vi "checkCalibrationChannel.vi"(8 "error in (no error)":errorcluster, 10 "Channel":T1, 11 "TEI9150 in":refnum<class "Tovey9150.lvclass">) -> (0 "error out":errorcluster, 2 "Items and Unit Numbers":string, 3 "TEI9150 out":refnum<class "Tovey9150.lvclass">)   [LabVIEW 2015, in "Tovey9150.lvclass"]
uses:
  Tovey9150.lvclass
  ToveyChannels.ctl
  Tovey9150.lvclass/Tovey9150.ctl
  <userlib>/Common/SerialProtocols/SerialCommunicator/SerialCommunicator.lvclass
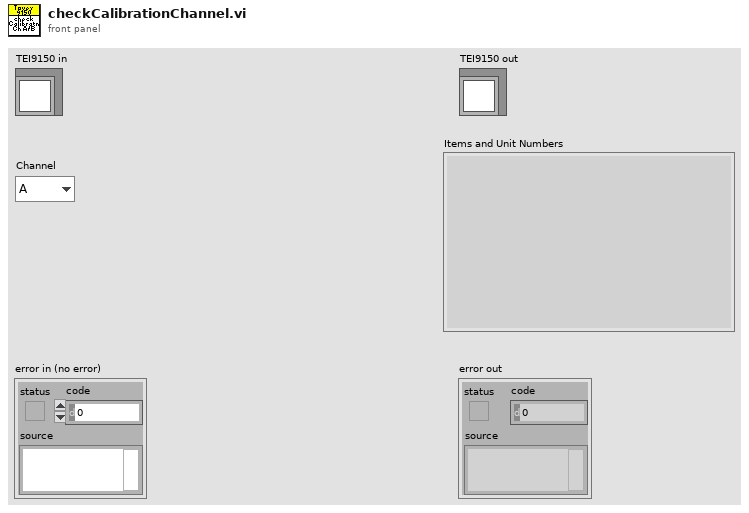
[diagram p1: front panel]
types:
  T1 = typedef "ToveyChannels.ctl" = enum16{"A", "B"}
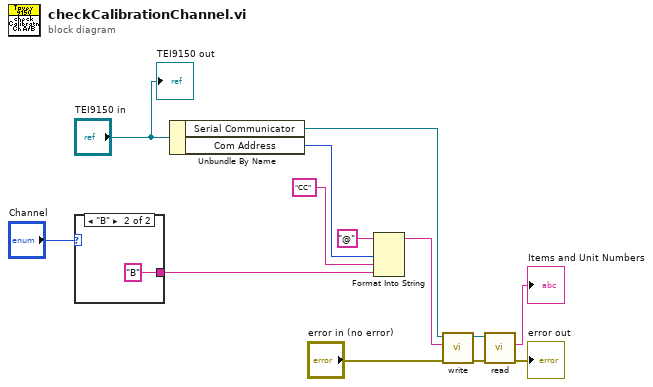
[diagram p0: block diagram]
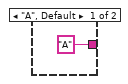
[diagram p2: hidden frame]
diagram:
  n1 = case shown="\"B\"" "Channel" {
    tunnel: ["A" "B"] -> w8
    frame "A", Default {
    }
    frame "B" {
    }
  }
  n2 = Unbundle By Name("TEI9150 in") -> ("Serial Communicator"=w5:refnum<class "SerialCommunicator.lvclass">, "Com Address"=w11:u8)
  n3 = Format Into String(initial string="@", w11, "CC" ("input 2"), w8) -> (resulting string=w4:string)  [unwired: 2 in, 1 out]
  n4 = call-dynamic "write.vi"("error in (no error)"="error in (no error)", "writeString"=w4, "SerialCommunicator in"=w5) -> ("error out"=w7:errorcluster, "SerialCommunicator out"=w6:refnum<class "SerialCommunicator.lvclass">)  [unwired: 7 in]
  n5 = call-dynamic "read.vi"("error in (no error)"=w7, "SerialCommunicator in"=w6) -> ("error out"=→"error out":errorcluster, "stringRead"=→"Items and Unit Numbers":string)  [unwired: 7 in, 1 out]
  "TEI9150 out" <- "TEI9150 in"
